vi "zad6.vi"() -> ()   [LabVIEW 2017]
panel:
  out "Array 2":dbl[](array[numeric])
  in  "Array":dbl[](array[numeric])
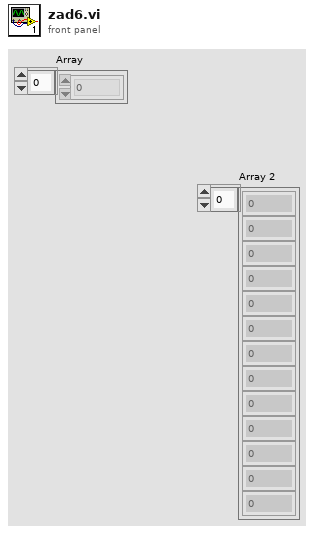
[diagram p1: front panel]
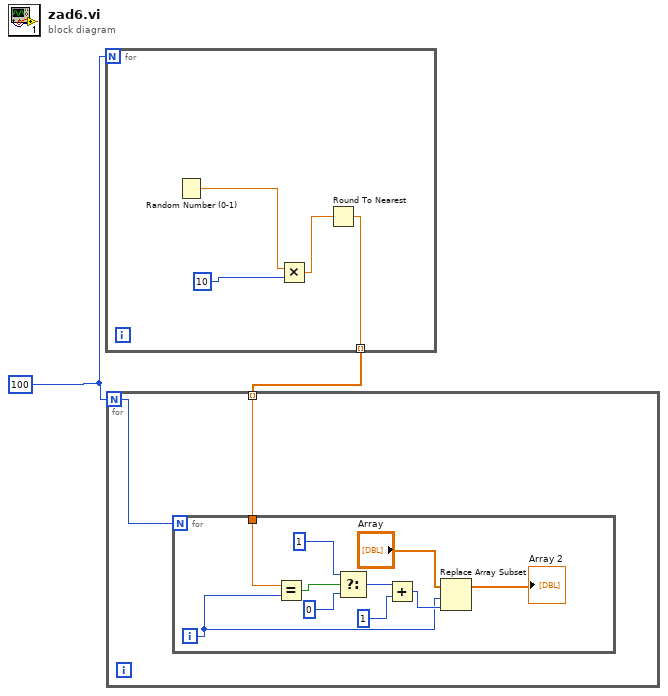
[diagram p0: block diagram]
diagram:
  w2 = u32 100 ("Numeric")
  n1 = for {
    N: w2 -> [_]
    tunnel: [w3] -> w1 mode=indexing
    n2 = Random Number (0-1)() -> (number: 0 to 1=w4:dbl)
    n3 = Multiply(x=w4, y=u32 10 ("Numeric")) -> (x*y=w6:dbl)
    n4 = Round To Nearest(number=w6) -> (nearest integer value=w3:dbl)
  }
  n5 = for {
    N: w2 -> [w8]
    tunnel: w1 -> [w7] mode=indexing
    n6 = for {
      N: w8 -> [_]
      tunnel: w7 -> [w18]
      i -> [w13]
      n7 = Equal?(x=w18, y=w13) -> (x = y?=w17:bool)
      n8 = Select(t=1, s=w17, f=0) -> (s? t:f=w15:i32)
      n9 = Add(x=w15, y=1) -> (x+y=w14:i32)
      n10 = Replace Array Subset(array="Array", new element=w14, index=w13) -> (→"Array 2":dbl[])
    }
  }
